vi "Launch UUDT Engine.vi"(8 "error in (no error)":errorcluster, 10 "Initial Parameters":T1(array[cluster]), 11 "VI Ref In":refnum<vi>) -> (0 "error out":errorcluster, 3 "VI Ref Out":refnum<vi>)   [LabVIEW 2019, in "GMLAN.lvlib"]
uses:
  GMLAN.lvlib
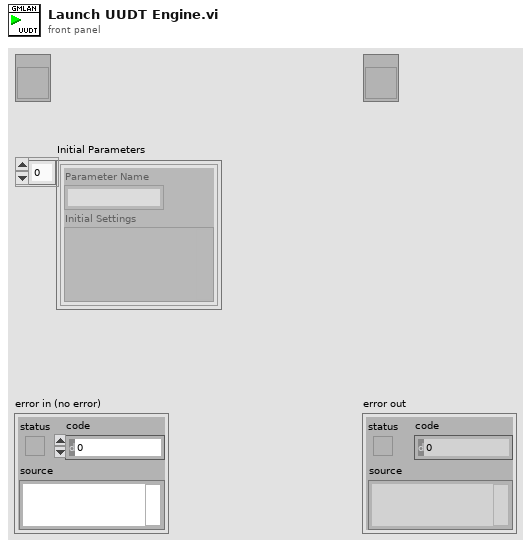
[diagram p1: front panel]
types:
  T1 = cluster{"Parameter Name":string, "Initial Settings":variant}[]
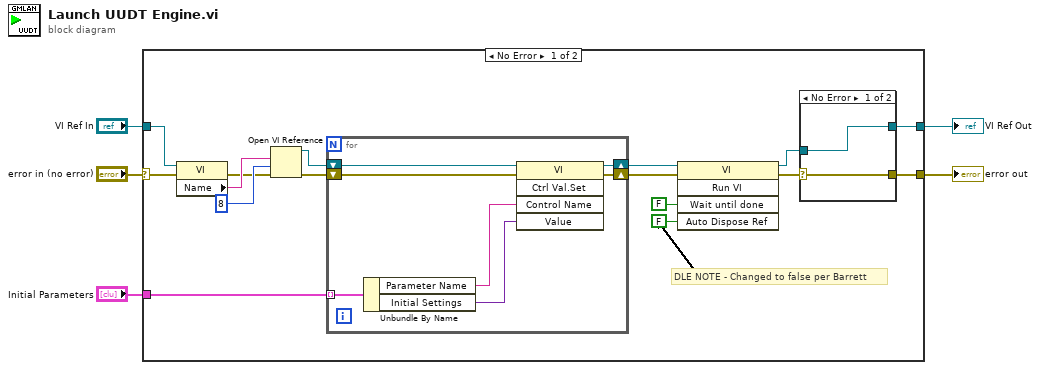
[diagram p0: block diagram]
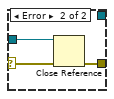
[diagram p2: hidden frame]
diagram:
  n1 = case shown="No Error" "error in (no error)" {
    selector: "error in (no error)" -> [w10 w35]
    tunnel: [w6 w35] -> w5
    tunnel: "VI Ref In" -> [w21 w34]
    tunnel: [w20 w34] -> w3
    tunnel: "Initial Parameters" -> [w7 _]
    frame No Error {
      # "DLE NOTE - Changed to false per Barrett"
      n2 = property class="VI"(reference=w21, error in=w10) -> (error out=w11:errorcluster, "Name"=w19:string)  [unwired: 1 out]
      n3 = Open VI Reference(vi path=w19, options=8, error in (no error)=w11) -> (vi reference=w8:refnum<vi>, error out=w9:errorcluster)  [unwired: 3 out]
      n4 = for {
        tunnel: w7 -> [w24] mode=indexing
        shift-right: [w27] -> w13
        shift-left: w8 -> [w25]
        shift-right: [w28] -> w14
        shift-left: w9 -> [w26]
        n5 = Unbundle By Name(w24) -> ("Parameter Name"=w23:string, "Initial Settings"=w22:variant)
        n6 = invoke class="VI" method="Ctrl Val.Set"(reference=w25, error in=w26, "Control Name"=w23, "Value"=w22) -> (reference out=w27:refnum<vi>, error out=w28:errorcluster)  [unwired: 1 in, 3 out]
      }
      n7 = invoke class="VI" method="Run VI"(reference=w13, error in=w14, "Wait until done"=FALSE ("Wait Until Done"), "Auto Dispose Ref"=FALSE ("Auto Dispose Reference")) -> (reference out=w15:refnum<vi>, error out=w16:errorcluster)  [unwired: 1 in, 3 out]
      n8 = case shown="No Error" w16 {
        selector: w16 -> [w30 w33]
        tunnel: w15 -> [w29 w32]
        tunnel: [w30 w31] -> w6
        tunnel: [w29 _] -> w20
        frame No Error {
        }
        frame Error {
          n9 = Close Reference(reference=w32, error in (no error)=w33) -> (error out=w31:errorcluster)
        }
      }
    }
    frame Error {
    }
  }
  "error out" <- w5
  "VI Ref Out" <- w3
